vi "Name_Script.vi"() -> (1 "StepScript":string="Sequence")   [LabVIEW 2016, in "SeqProcessor.lvlib"]
uses:
  SeqProcessor.lvlib
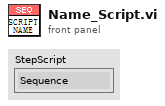
[diagram p1: front panel]
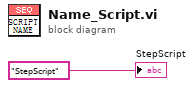
[diagram p0: block diagram]
diagram:
  "StepScript" <- "StepScript" ("Tag")
